vi "Precedence.vi"(11 "Token Type":T1) -> (3 "Precedence":u8)   [LabVIEW 2022 SP3, in "Pipes.lvlib"]
uses:
  Controls/Token Type.ctl
  Pipes.lvlib
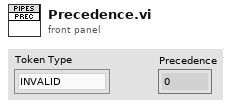
[diagram p1: front panel]
types:
  T1 = typedef "Pipes.lvlib/Token Type.ctl" = enum8{"INVALID", "NOT", "AND", "OR", "EE", "NE", "LT", "GT", "LTE", "GTE", "PLUS", "MINUS", "MULTIPLY", "DIVIDE", "MODULUS", "LPAREN", "RPAREN", "LITERAL", "IDENTIFIER", "DEFINITION"}
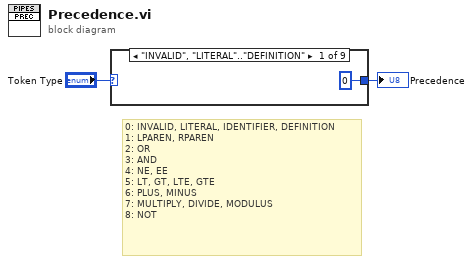
[diagram p0: block diagram]
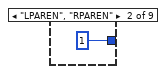
[diagram p2: hidden frame]
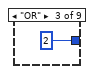
[diagram p3: hidden frame]
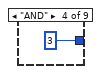
[diagram p4: hidden frame]
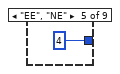
[diagram p5: hidden frame]
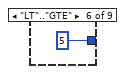
[diagram p6: hidden frame]
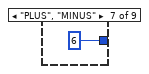
[diagram p7: hidden frame]
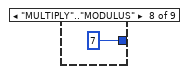
[diagram p8: hidden frame]
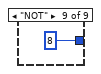
[diagram p9: hidden frame]
diagram:
  # "0: INVALID, LITERAL, IDENTIFIER, DEFINITION\n1: LPAREN, RPAREN\n2: OR\n3: AND\n4: NE, EE\n5: LT, GT, LTE, GTE\n6: PLUS, MINUS\n7: MULTIPLY, DIVIDE, MODULUS\n8: NOT"
  n1 = case shown="\"INVALID\", \"LITERAL\"..\"DEFINITION\"" "Token Type" {
    tunnel: [u8 0 ("Precedence") u8 1 ("Precedence") u8 2 ("Precedence") u8 3 ("Precedence") u8 4 ("Precedence") u8 5 ("Precedence") u8 6 ("Precedence") u8 7 ("Precedence") u8 8 ("Precedence")] -> w1
    frame "INVALID", "LITERAL".."DEFINITION" {
    }
    frame "LPAREN", "RPAREN" {
    }
    frame "OR" {
    }
    frame "AND" {
    }
    frame "EE", "NE" {
    }
    frame "LT".."GTE" {
    }
    frame "PLUS", "MINUS" {
    }
    frame "MULTIPLY".."MODULUS" {
    }
    frame "NOT" {
    }
  }
  "Precedence" <- w1
